vi "Write Command _Arm_.vi"(8 "error in (no error)":errorcluster, 10 "Command \"Arm\"":string, 11 "SupplyControl in":refnum<class "SupplyControl.lvclass">) -> (0 "error out":errorcluster, 3 "SupplyControl out":refnum<class "SupplyControl.lvclass">)   [LabVIEW 2018, in "SupplyControl.lvclass"]
uses:
  SupplyControl.lvclass
  SupplyControl.lvclass/SupplyControl.ctl
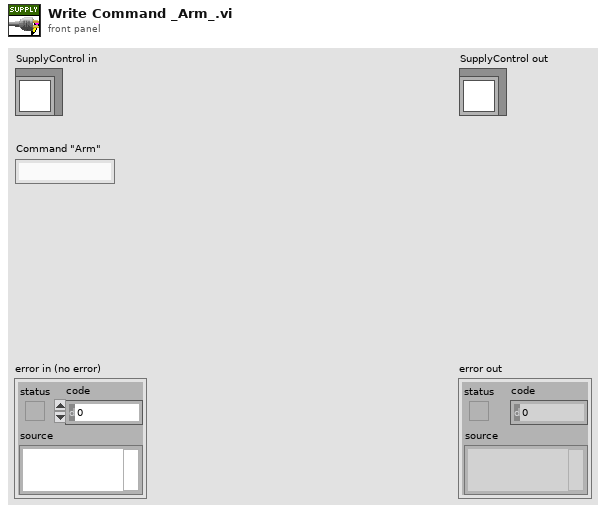
[diagram p1: front panel]
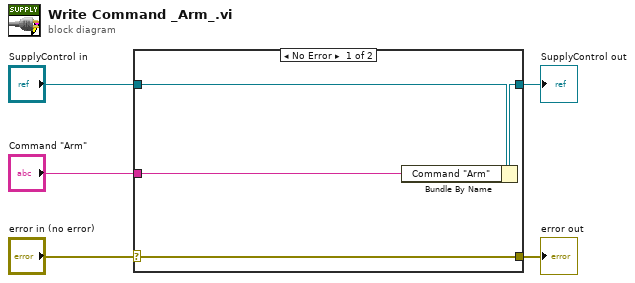
[diagram p0: block diagram]
diagram:
  n1 = case shown="No Error" "error in (no error)" {
    selector: "error in (no error)" -> [w9 w10]
    tunnel: [w9 w10] -> w4
    tunnel: [w7 w11] -> w2
    tunnel: "SupplyControl in" -> [w8 w11]
    tunnel: "Command \"Arm\"" -> [w6 _]
    frame No Error {
      n2 = Bundle By Name(cluster=w8, "Command \"Arm\""=w6) -> (w7:refnum<class "SupplyControl.lvclass">)
    }
    frame Error {
    }
  }
  "error out" <- w4
  "SupplyControl out" <- w2
